vi "Init.vi"(7 "Enqueuer in":refnum<class "Message Enqueuer.lvclass">, 8 "error in (no error)":errorcluster, 9 "mode":T1, 10 "common":T2={"id"="", "threshold"=enum."INFO", "filter"={"mode"=enum."Mirror", "levelMin"=enum."INFO", "levelMax"=enum."INFO", "tagPrefix"=""}, "queueBound"=-1, "dropPolicy"=enum."DropOldest", "useUTC"=FALSE}, 11 "RelayAppender in":refnum<class "RelayAppender.lvclass">) -> (0 "error out":errorcluster, 3 "RelayAppender out":refnum<class "RelayAppender.lvclass">)   [LabVIEW 2026, in "Lumberjack.lvlib" / "RelayAppender.lvclass"]
doc: "Stamps a RelayAppenderConfig into the relay appender and, in queue mode, creates its named relay queue.\nCalls the common Init (InitCommon) for the shared gate/config, derives the queue name from the appender id (RelayQueueName), and obtains the relay queue so the application can drain it; message-mode relays deliver via the consumer enqueuer instead (SRS-LMBR-025).\nLumberjack.lvlib, RelayAppender.lvclass, public."
uses:
  RelayAppender.lvclass
  TypeDefs/AppenderConfig.ctl
  TypeDefs/Severity.ctl
  TypeDefs/Filter.ctl
  TypeDefs/FilterMode.ctl
  TypeDefs/DropPolicy.ctl
  TypeDefs/RelayMode.ctl
  <vilib>/ActorFramework/Message Enqueuer/Message Enqueuer.lvclass
  RelayAppender.lvclass/RelayAppender.ctl
  TypeDefs/Statement.ctl
  Appender.lvclass/Appender.lvclass
  Lumberjack.lvlib
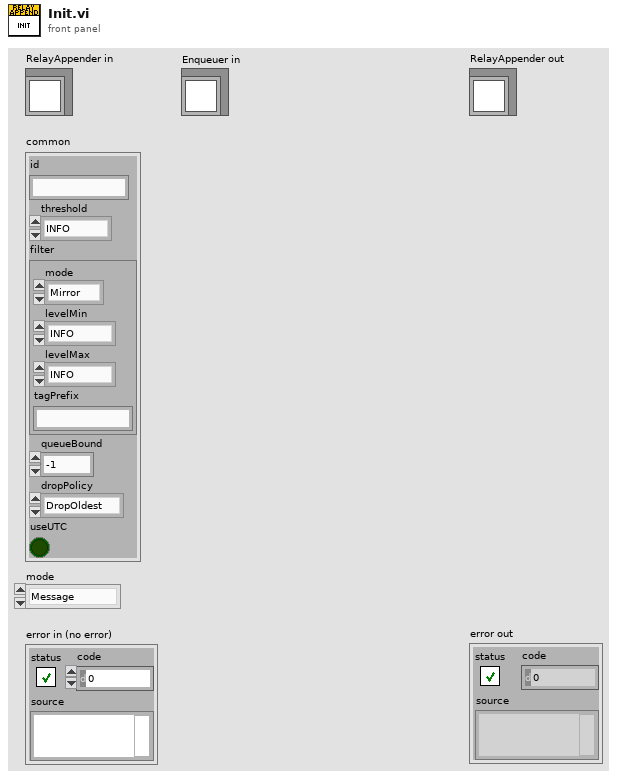
[diagram p1: front panel]
types:
  T1 = typedef "Lumberjack.lvlib/RelayMode.ctl" = enum16{"Message", "Queue"}
  T2 = typedef "Lumberjack.lvlib/AppenderConfig.ctl" = cluster{"id":string, "threshold":T3, "filter":T4, "queueBound":i32, "dropPolicy":T6, "useUTC":bool}
  T3 = typedef "Lumberjack.lvlib/Severity.ctl" = enum16{"OFF", "FATAL", "ERROR", "WARN", "INFO", "DEBUG", "TRACE", "ALL"}
  T4 = typedef "Lumberjack.lvlib/Filter.ctl" = cluster{"mode":T5, "levelMin":T3, "levelMax":T3, "tagPrefix":string}
  T5 = typedef "Lumberjack.lvlib/FilterMode.ctl" = enum16{"Mirror", "Routed"}
  T6 = typedef "Lumberjack.lvlib/DropPolicy.ctl" = enum16{"DropOldest", "DropNewest", "LevelAware"}
  T7 = typedef "Lumberjack.lvlib/Statement.ctl" = cluster{"timestamp":timestamp, "level":T3, "sourceTag":string, "originVI":string, "message":string}
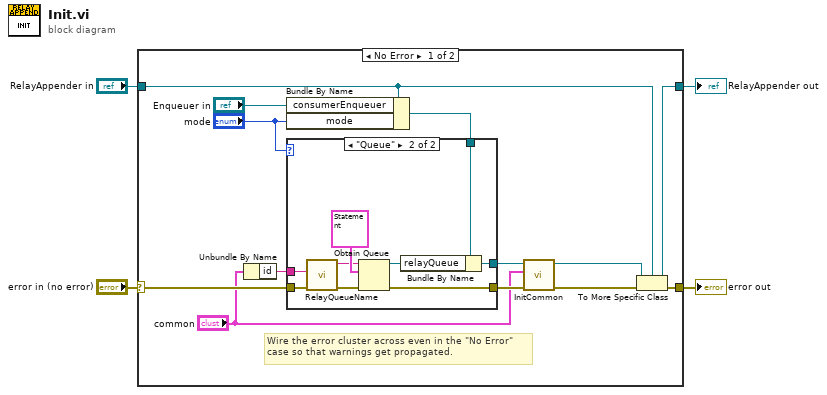
[diagram p0: block diagram]
diagram:
  n1 = case shown="No Error" "error in (no error)" {
    selector: "error in (no error)" -> [w17 w30]
    tunnel: [w10 w30] -> w3
    tunnel: [w7 w29] -> w1
    tunnel: "RelayAppender in" -> [w9 w29]
    frame No Error {
      # "Wire the error cluster across even in the \"No Error\"\ncase so that warnings get propagated."
      n2 = Unbundle By Name("common") -> ("id"=w5:string)
      n3 = Bundle By Name(cluster=w9, "consumerEnqueuer"="Enqueuer in", "mode"="mode") -> (w13:refnum<class "RelayAppender.lvclass">)
      n4 = case shown="\"Queue\"" "mode" {
        tunnel: w17 -> [w19 w23]
        tunnel: [w19 w28] -> w14
        tunnel: w13 -> [w18 w27]
        tunnel: [w18 w24] -> w12
        tunnel: w5 -> [_ w22]
        frame "Message", Default {
        }
        frame "Queue" {
          n5 = call "RelayQueueName.vi"("error in (no error)"=w23, "id"=w22) -> ("error out"=w20:errorcluster, "queueName"=w21:string)  [unwired: 8 in]
          n6 = Obtain Queue(name (unnamed)=w21, element data type=T7 {"timestamp"=timestamp(0 s since 1904-01-01), "level"=enum."INFO", "sourceTag"="", "originVI"="", "message"=""} ("Statement"), error in (no error)=w20) -> (queue out=w26:refnum<queue>, error out=w28:errorcluster)  [unwired: 2 in, 1 out]
          n7 = Bundle By Name(cluster=w27, "relayQueue"=w26) -> (w24:refnum<class "RelayAppender.lvclass">)
        }
      }
      n8 = call "InitCommon.vi"("error in (no error)"=w14, "AppenderConfig"="common", "Appender in"=w12) -> ("error out"=w11:errorcluster, "Appender out"=w8:refnum<class "RelayAppender.lvclass">)  [unwired: 7 in]
      n9 = To More Specific Class(target class=w9, reference=w8, error in=w11) -> (specific class reference=w7:refnum<class "RelayAppender.lvclass">, error out=w10:errorcluster)
    }
    frame Error {
    }
  }
  "error out" <- w3
  "RelayAppender out" <- w1
